vi "Message type.vi"(7 "E&S Message":T2, 9 "error in (no error)":errorcluster) -> (2 "Elevated priority":bool, 6 "Type":T1, 8 "Content":variant, 10 "error out":errorcluster)   [LabVIEW 2011]
uses:
  emi Lib/System 01/0 - General/S&E reporting/Private/_emi_ S&E Message.ctl
  emi Lib/System 01/0 - General/S&E reporting/Private/_emi_ S&E Message type.ctl
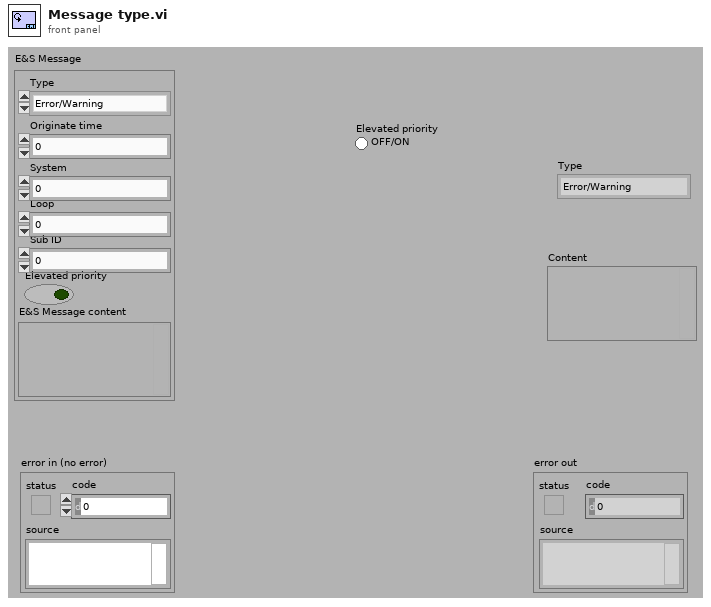
[diagram p1: front panel]
types:
  T1 = typedef "_emi_ S&E Message type.ctl" = enum16{"Error/Warning", "Note", "Debug", "Event", "Alarm Analog", "Alarm Digital", "Annotation"}
  T2 = typedef "_emi_ S&E Message.ctl" = cluster{"Type":T1, "Originate time":dbl, "System":u8, "Loop":u16, "Sub ID":u16, "Elevated priority":bool, "E&S Message content":variant}
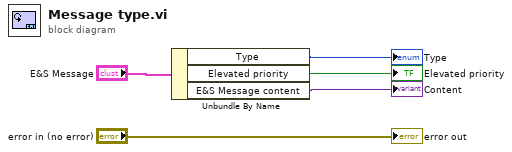
[diagram p0: block diagram]
diagram:
  n1 = Unbundle By Name("E&S Message") -> ("Type"=→"Type":T1, "Elevated priority"=→"Elevated priority":bool, "E&S Message content"=→"Content":variant)
  "error out" <- "error in (no error)"
